vi "tiffOpenForWrite.vi"(11 "Path":path) -> (3 "TiffOut":refnum<k24>)   [LabVIEW 2018, in "LVTiffWriter.lvlib"]
doc: "Opens file for writing tiffs."
uses:
  LVTiffWriter.lvlib
  C:/Users/johan/Downloads/LabVIEW software/LabVIEW software/IX-81 Software/lib/tiff/LVTiffWriter/BitMiracle.LibTiff.NET.dll
  BitMiracle.LibTiff.NET.dll
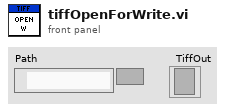
[diagram p1: front panel]
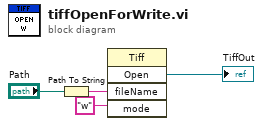
[diagram p0: block diagram]
diagram:
  n1 = Path To String(path="Path") -> (string=w4:string)
  n2 = invoke class="Tiff" method="Open"("fileName"=w4, "mode"="w") -> ("Open"=→"TiffOut":refnum<k24>)  [unwired: 3 in, 4 out]
